vi "Trajectory_Controller.vi"(0 "Error In":errorcluster, 1 "reset":dbl, 5 "Configuration":T1={"Accelerometer Bias"={"X (m/s)"=0.0, "Y (m/s)"=0.0, "Z (m/s)"=0.0}, "Gyroscope Bias"={"X (m/s)"=0.0, "Y (m/s)"=0.0, "Z (m/s)"=0.0}, "Steering Motor Gear Ratio"=611.0, "Steering Pully Gear Ratio"=1.0, "Steering Encoder CPR"=500.0, "Steering Motor Max RPM"=4000.0, "Wheelbase (m)"=1.12, "Fork Angle (rad)"=1.3, "Balancing Controller"={"Kp (/s)"=1.0, "Kd (1)"=1.0}, "Max Allowed Steering Angle (rad)"=0.7, "Task Periods"={"Emergency Stop (us)"=10000, "IMU (us)"=10000, "Steering Motor Encoder (us)"=10000, "State Estimator (us)"=10000, "Balancing Controller (us)"=10000, "GNSS (us)"=10000, "Logging (us)"=50000, "Drive Motor (us)"=100000}, "Drive Motor Gear Ratio"=0.7, "lr"=0.0, "lf"=0.0, "lambda"=0.0, "k1"=0.0, "k2"=0.0, "e1_max"=0.0, "Ad_t"=0.0, "Bd_t"=0.0, "C_t"=0.0, "D_t"=0.0, "Wheel radius"=0.311}, 7 "State Estimate In":refnum<data-value>, 9 "Reset and Init trajectory":bool, 11 "RefTraj in":refnum<data-value>, 12 "Trajectory In":refnum<data-value>, 13 "Measurement In":refnum<data-value>) -> (2 "Measurement Out":refnum<data-value>, 6 "Error out":errorcluster, 10 "Trajectory Out":refnum<data-value>)   [LabVIEW 2021]
uses:
  State Estimator/State Estimate.ctl
  Trajectory_Control.ctl
  Configuration/Configuration.ctl
  State Estimator/Measurements.ctl
  IMU/IMU Data.ctl
  Steering Motor Encoder/Steering Motor Encoder Data.ctl
  GNSS/GNSS Data.ctl
panel:
  out "State Estimate In 2":refnum<data-value>
  out "RefTraj out":refnum<data-value>
  out "size(s)":i32[](array[numeric])
  out "error2":dbl
  out "error1":dbl
  out "Rollref":dbl
  out "Closestpoint":dbl
  in  "path in":path=path "libtrajectory_controller.so"
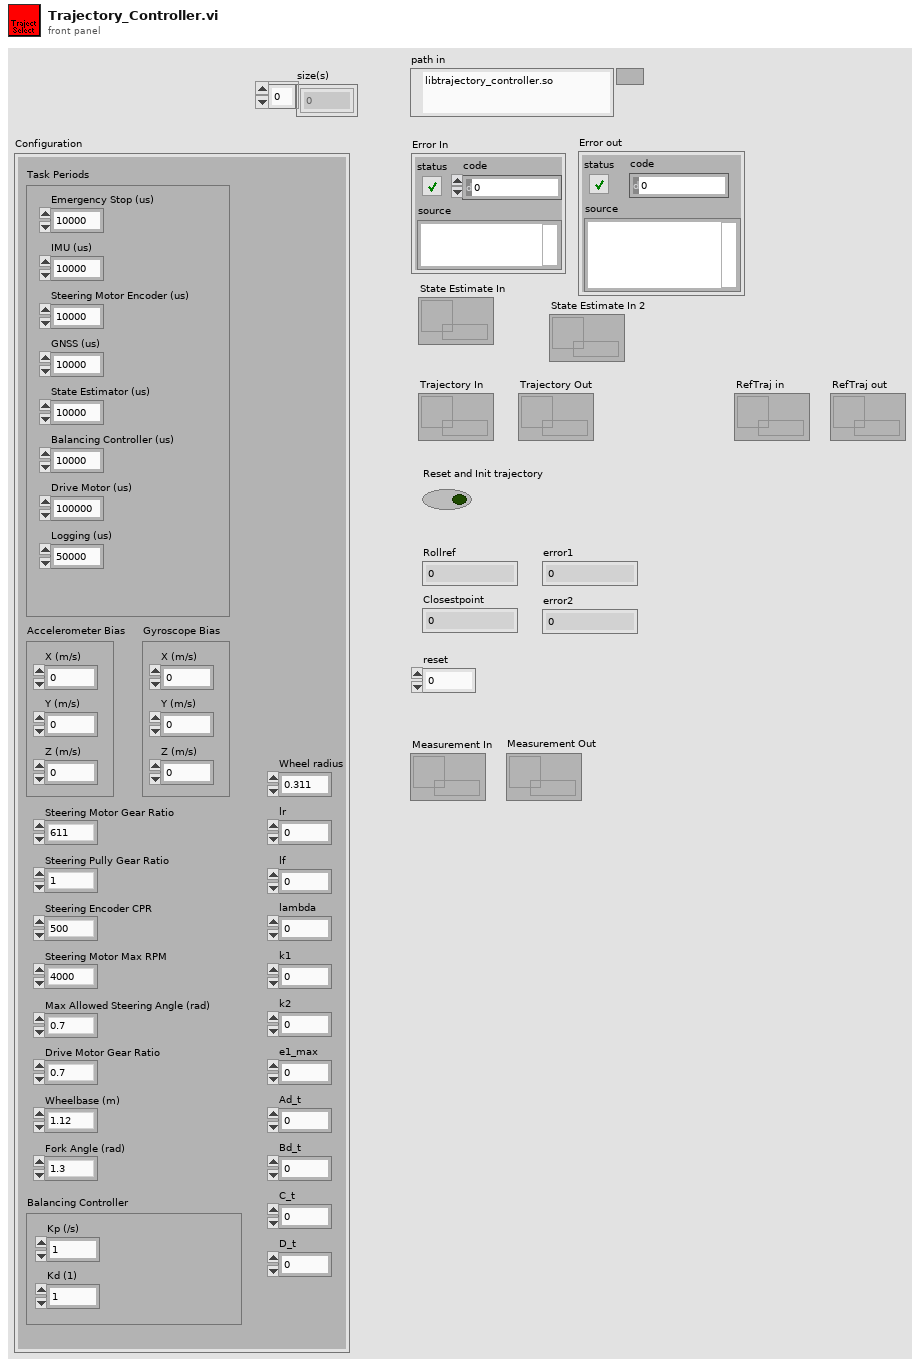
[diagram p1: front panel]
types:
  T1 = typedef "Configuration.ctl" = cluster{"Accelerometer Bias":cluster{"X (m/s)":dbl, "Y (m/s)":dbl, "Z (m/s)":dbl}, "Gyroscope Bias":cluster{"X (m/s)":dbl, "Y (m/s)":dbl, "Z (m/s)":dbl}, "Steering Motor Gear Ratio":dbl, "Steering Pully Gear Ratio":dbl, "Steering Encoder CPR":dbl, "Steering Motor Max RPM":dbl, "Wheelbase (m)":dbl, "Fork Angle (rad)":dbl, "Balancing Controller":cluster{"Kp (/s)":dbl, "Kd (1)":dbl}, "Max Allowed Steering Angle (rad)":dbl, "Task Periods":cluster{"Emergency Stop (us)":i64, "IMU (us)":i64, "Steering Motor Encoder (us)":i64, "State Estimator (us)":i64, "Balancing Controller (us)":i64, "GNSS (us)":i64, "Logging (us)":i64, "Drive Motor (us)":i64}, "Drive Motor Gear Ratio":dbl, "lr":dbl, "lf":dbl, "lambda":dbl, "k1":dbl, "k2":dbl, "e1_max":dbl, "Ad_t":dbl, "Bd_t":dbl, "C_t":dbl, "D_t":dbl, "Wheel radius":dbl}
  T2 = typedef "Trajectory_Control.ctl" = cluster{"Rollref":dbl, "Closestpoint":dbl, "Error1":dbl, "Error2":dbl, "Dpsiref_cont":dbl, "Lateral_cont":dbl, "Heading_cont":dbl, "Reset_traj":dbl}
  T3 = typedef "Measurements.ctl" = cluster{"IMU Data":T4, "Steering Motor Encoder Data":T5, "GNSS Data":T6}
  T4 = typedef "IMU Data.ctl" = cluster{"Gyroscope":cluster{"X (rad/s)":dbl, "Y (rad/s)":dbl, "Z (rad/s)":dbl}, "Accelerometer":cluster{"X (m/s^2)":dbl, "Y (m/s^2)":dbl, "Z (m/s^2)":dbl}, "Flag IMU":dbl}
  T5 = typedef "Steering Motor Encoder Data.ctl" = cluster{"Encoder Position (counts)":i32, "Steering Angle (rad)":dbl, "Flag Steering Encoder":dbl}
  T6 = typedef "GNSS Data.ctl" = cluster{"Latitude (rad)":dbl, "Longitude (rad)":dbl, "Altitude (m)":dbl, "Speed (m/s)":dbl, "Heading (rad)":dbl, "Fix Quality":i32, "Number of Satellites":i32, "Latitude (deg)":dbl, "Longitude (deg)":dbl, "Flag GNSS":dbl}
  T7 = typedef "State Estimate.ctl" = cluster{"X (m)":dbl, "Y (m)":dbl, "Psi (rad)":dbl, "Roll (rad)":dbl, "Roll Rate (rad/s)":dbl, "delta":dbl, "velocity":dbl}
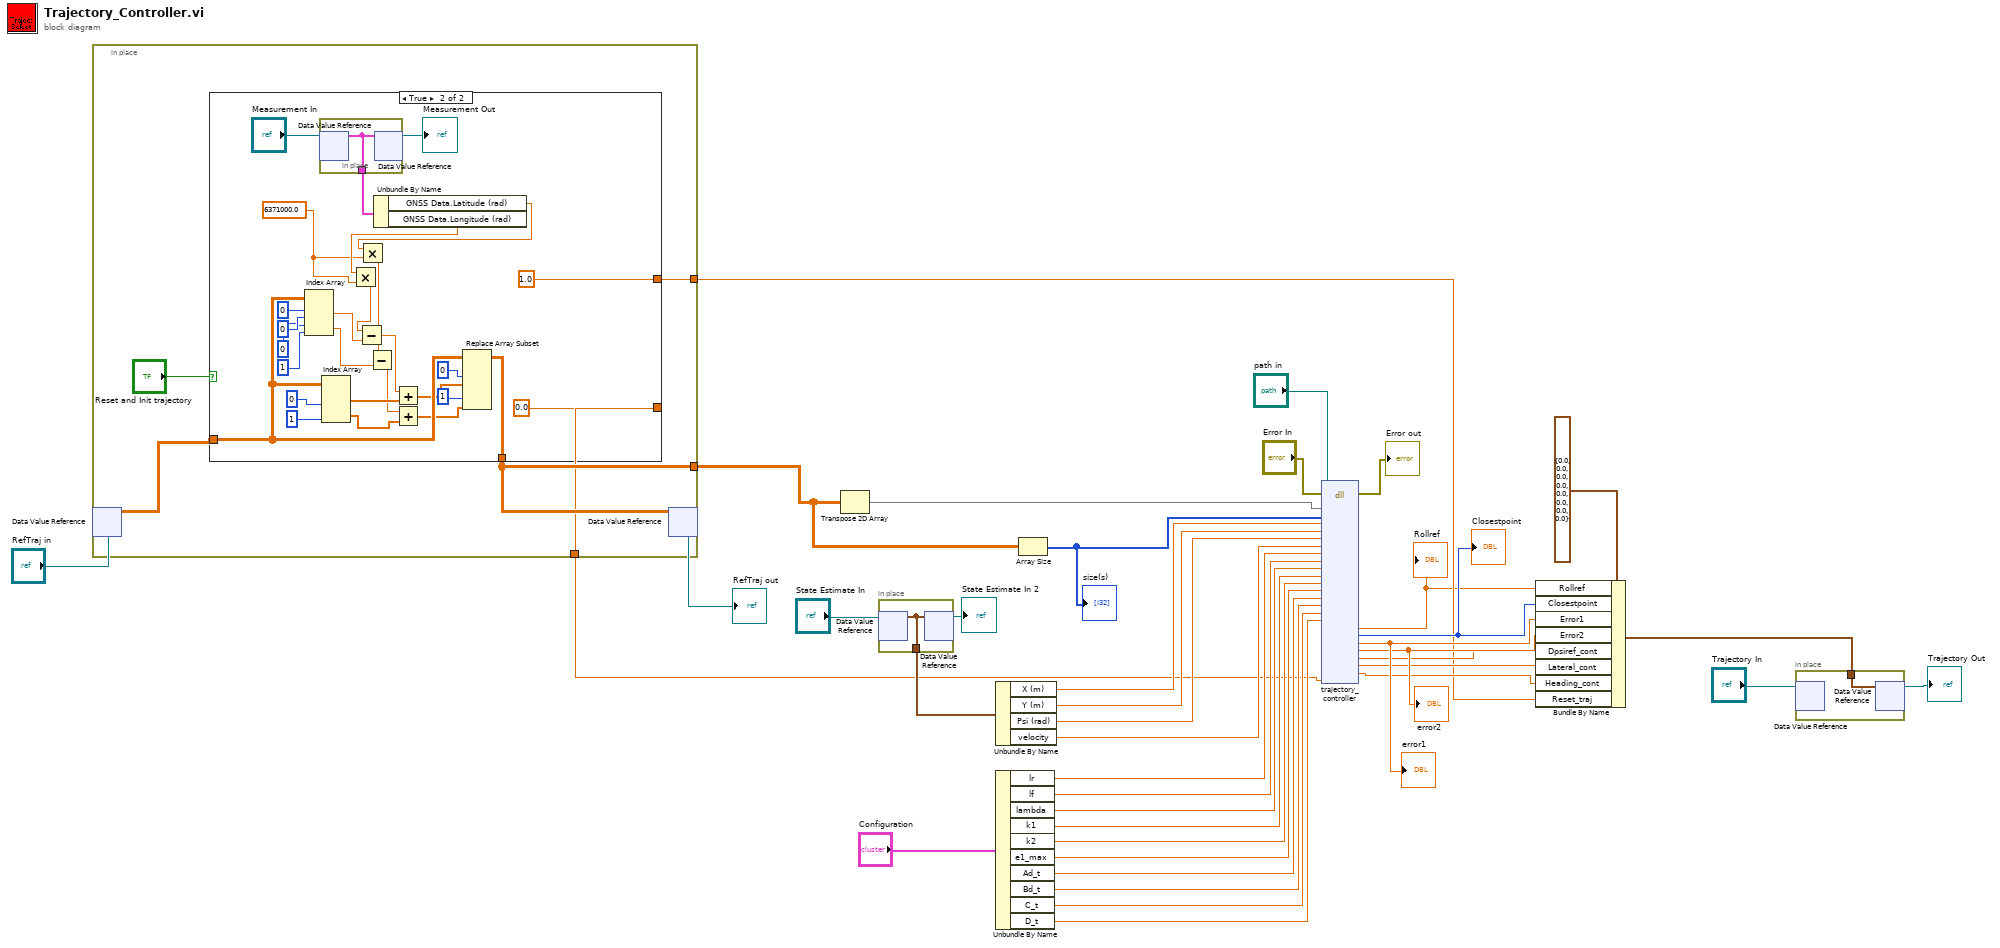
[diagram p0: block diagram]
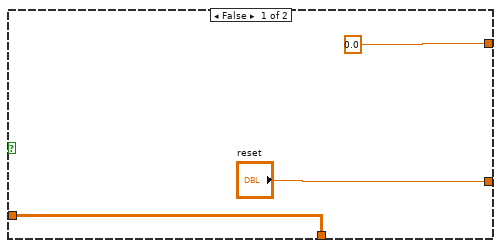
[diagram p2: hidden frame]
diagram:
  n1 = in-place {
    in-place-border: [w42] -> w2
    in-place-border: [w44] -> w5
    in-place-border: [w40] -> w4
    n2 = in-place-dvr #1("RefTraj in") -> (w43:dbl[][])  [unwired: 1 out]
    n3 = case shown="True" "Reset and Init trajectory" {
      tunnel: ["reset" 0.0] -> w42
      tunnel: [w46 w53] -> w44
      tunnel: w43 -> [w46 w64]
      tunnel: [0.0 1.0] -> w40
      frame False {
      }
      frame True {
        w67 = 6371000.0
        n4 = Index Array(array=w64, index (row) #1=0, index (col) #1=0, index (row) #2=0, index (col) #2=1) -> (element #1=w59:dbl, element #2=w58:dbl)
        n5 = in-place {
          in-place-border: [w76] -> w72
          n6 = in-place-dvr #2("Measurement In") -> (w76:T3)  [unwired: 1 out]
          n7 = in-place-dvr #2(w76) -> (→"Measurement Out":refnum<data-value>)  [unwired: 1 out]
        }
        n8 = Index Array(array=w64, index (col) #1=0, index (col) #2=1) -> (element #1=w70:dbl[], element #2=w55:dbl[])  [unwired: 2 in]
        n9 = Unbundle By Name(w72) -> ("GNSS Data.Latitude (rad)"=w69:dbl, "GNSS Data.Longitude (rad)"=w68:dbl)
        n10 = Multiply(x=w68, y=w67) -> (x*y=w65:dbl)
        n11 = Subtract(x=w65, y=w59) -> (x-y=w71:dbl)
        n12 = Multiply(x=w69, y=w67) -> (x*y=w66:dbl)
        n13 = Subtract(x=w66, y=w58) -> (x-y=w56:dbl)
        n14 = Add(x=w71, y=w70) -> (x+y=w57:dbl[])
        n15 = Add(x=w56, y=w55) -> (x+y=w54:dbl[])
        n16 = Replace Array Subset(array=w64, new element #1=w57, index (col) #1=0, new element #2=w54, index (col) #2=1) -> (w53:dbl[][])  [unwired: 2 in]
      }
    }
    n17 = in-place-dvr #1(w44) -> (→"RefTraj out":refnum<data-value>)  [unwired: 1 out]
  }
  n18 = Transpose 2D Array(2D array=w5) -> (transposed array=w6:dbl[][])
  n19 = in-place {
    in-place-border: [w77] -> w37
    n20 = in-place-dvr #3("State Estimate In") -> (w77:T7)  [unwired: 1 out]
    n21 = in-place-dvr #3(w77) -> (→"State Estimate In 2":refnum<data-value>)  [unwired: 1 out]
  }
  n22 = Unbundle By Name(w37) -> ("X (m)"=w36:dbl, "Y (m)"=w35:dbl, "Psi (rad)"=w34:dbl, "velocity"=w17:dbl)
  n23 = Unbundle By Name("Configuration") -> ("lr"=w27:dbl, "lf"=w26:dbl, "lambda"=w25:dbl, "k1"=w24:dbl, "k2"=w23:dbl, "e1_max"=w22:dbl, "Ad_t"=w21:dbl, "Bd_t"=w20:dbl, "C_t"=w19:dbl, "D_t"=w18:dbl)
  n24 = Array Size(array=w5) -> (size(s)=w7:i32[])
  "size(s)" <- w7
  n25 = dll-call lib="libtrajectory_controller.so" fn="trajectory_controller"(path in="path in", error in="Error In", "Traj"=w6, "traj_size"=w7, "X"=w36, "Y"=w35, "Psi"=w34, "v"=w17, "lr"=w27, "lf"=w26, "lambda"=w25, "k1"=w24, "k2"=w23, "e1max"=w22, "Adt"=w21, "Bdt"=w20, "Ct"=w19, "Dt"=w18, "Reset"=w2) -> (error out=→"Error out":errorcluster, "Rollref"=w1:dbl, "Closestpoint"=w13:i32, "error1"=w15:dbl, "error2"=w14:dbl, "dpsiref_cont"=w12:dbl, "Lateral_cont"=w11:dbl, "Heading_cont"=w10:dbl)  [unwired: 26 in, 1 out]
  "Closestpoint" <- w13
  "Rollref" <- w1
  "error1" <- w15
  "error2" <- w14
  n26 = Bundle By Name(cluster=T2 {"Rollref"=0.0, "Closestpoint"=0.0, "Error1"=0.0, "Error2"=0.0, "Dpsiref_cont"=0.0, "Lateral_cont"=0.0, "Heading_cont"=0.0, "Reset_traj"=0.0} ("Trajectory (Debug)"), "Rollref"=w1, "Closestpoint"=w13, "Error1"=w15, "Error2"=w14, "Dpsiref_cont"=w12, "Lateral_cont"=w11, "Heading_cont"=w10, "Reset_traj"=w4) -> (w29:T2)
  n27 = in-place {
    in-place-border: w29 -> [w78]
    n28 = in-place-dvr #4("Trajectory In") -> ()  [unwired: 2 out]
    n29 = in-place-dvr #4(w78) -> (→"Trajectory Out":refnum<data-value>)  [unwired: 1 out]
  }
